vi "INSTRUMENTORDERSVotageAC5_6.vi"(0 "VISA资源名称":refnum<visa-resource-name>="DPO5054-C012667", 1 "打开通道":u16(ring) items=["CH1", "CH2", "CH3", "CH4"], 2 "关闭通道":u16(ring) items=["CH1", "CH2", "CH3", "CH4"], 3 "行索引":i32, 5 "错误输入（无错误）":errorcluster) -> (11 "FREQ":dbl, 13 "PERIOD":dbl, 14 "RMS":dbl, 15 "AMP":dbl, 16 "MAX":dbl, 17 "MIN":dbl, 18 "PK2PK":dbl, 19 "错误输出":errorcluster)   [LabVIEW 2014]
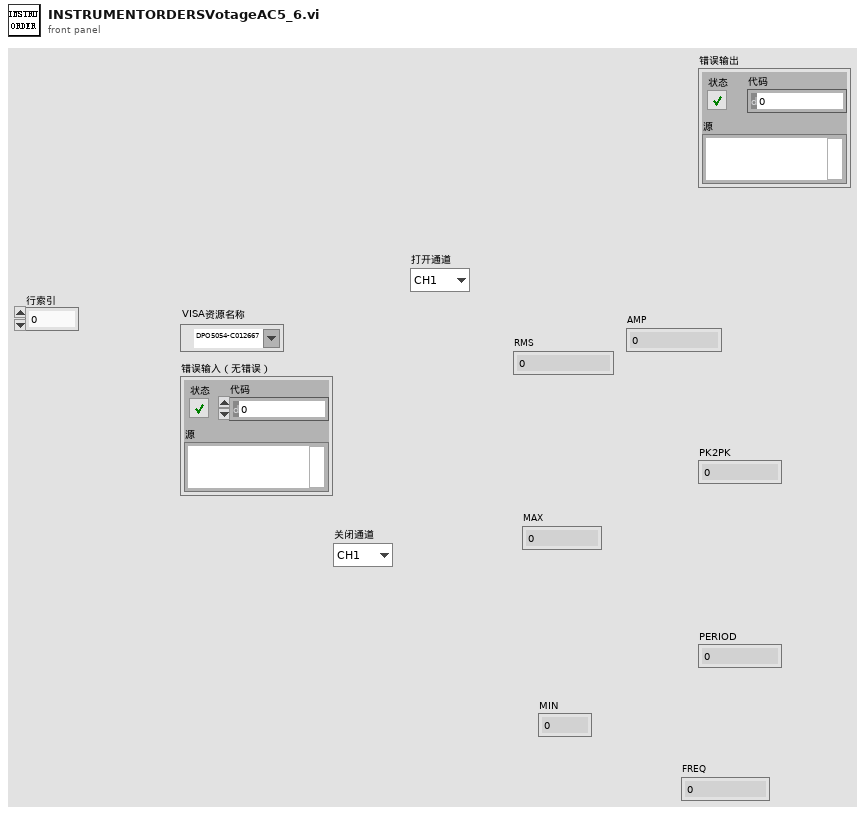
[diagram p1: front panel]
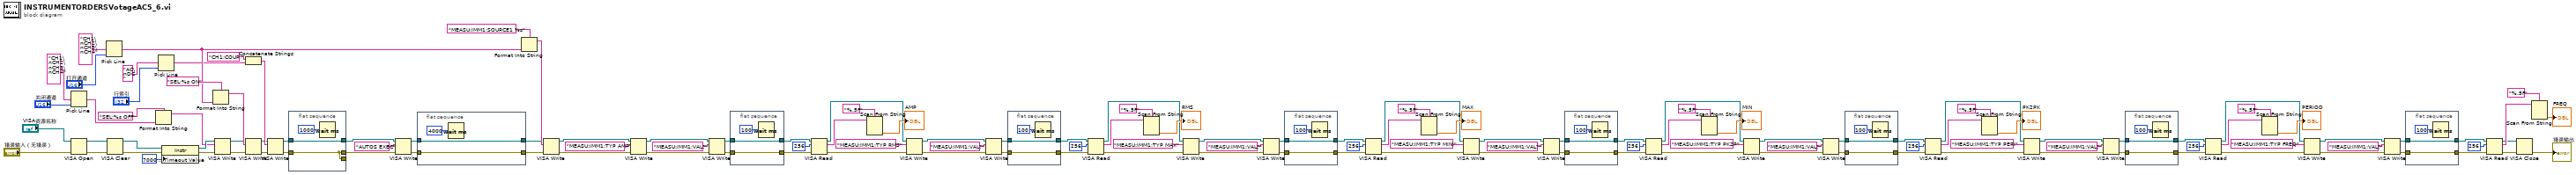
[diagram p0: block diagram]
diagram:
  n1 = Pick Line(multi-line string="CH1\nCH2\nCH3\nCH4" ("多行字符串"), line index="关闭通道") -> (output string=w113:string)  [unwired: 1 in]
  n2 = VISA Open(error in (no error)="错误输入（无错误）", VISA resource name="VISA资源名称") -> (VISA resource name=w139:refnum<visa-resource-name>, error out=w138:errorcluster)  [unwired: 3 in]
  n3 = Pick Line(multi-line string="CH1\nCH2\nCH3\nCH4" ("多行字符串"), line index="打开通道") -> (output string=w118:string)  [unwired: 1 in]
  n4 = VISA Clear(VISA resource name=w139, error in (no error)=w138) -> (VISA resource name out=w137:refnum<visa-resource-name>, error out=w136:errorcluster)
  n5 = Format Into String(format string="SEL:%s OFF" ("格式字符串"), w113) -> (resulting string=w109:string)  [unwired: 2 in, 1 out]
  n6 = Pick Line(multi-line string="AC\nDC", line index="行索引") -> (output string=w12:string)  [unwired: 1 in]
  n7 = property class="Instr"(reference=w137, error in=w136, "General Settings:Timeout Value"=u32 7000) -> (reference out=w115:refnum<visa-resource-name>, error out=w114:errorcluster)
  n8 = Format Into String(format string="SEL:%s ON" ("格式字符串"), w118) -> (resulting string=w117:string)  [unwired: 2 in, 1 out]
  n9 = VISA Write(VISA resource name=w115, write buffer=w109, error in (no error)=w114) -> (VISA resource name out=w108:refnum<visa-resource-name>, error out=w107:errorcluster)  [unwired: 1 out]
  n10 = Concatenate Strings("CH1:COUP " ("写入缓冲区"), w12) -> (w11:string)
  n11 = VISA Write(VISA resource name=w108, write buffer=w117, error in (no error)=w107) -> (VISA resource name out=w10:refnum<visa-resource-name>, error out=w9:errorcluster)  [unwired: 1 out]
  n12 = VISA Write(VISA resource name=w10, write buffer=w11, error in (no error)=w9) -> (VISA resource name out=w4:refnum<visa-resource-name>, error out=w3:errorcluster)  [unwired: 1 out]
  n13 = flat-sequence {
    tunnel: w4 -> [w142]
    tunnel: [w142] -> w2
    tunnel: w3 -> [w141]
    tunnel: [w141] -> _
    tunnel: [w141] -> w1
    frame #0 {
      n14 = Wait (ms)(milliseconds to wait=u32 1000 ("等待时间（毫秒）")) -> ()  [unwired: 1 out]
    }
  }
  n15 = VISA Write(VISA resource name=w2, write buffer="AUTOS EXEC" ("写入缓冲区"), error in (no error)=w1) -> (VISA resource name out=w8:refnum<visa-resource-name>, error out=w7:errorcluster)  [unwired: 1 out]
  n16 = flat-sequence {
    tunnel: w8 -> [w145]
    tunnel: [w145] -> w6
    tunnel: w7 -> [w144]
    tunnel: [w144] -> w5
    frame #0 {
      n17 = Wait (ms)(milliseconds to wait=u32 4000 ("等待时间（毫秒）")) -> ()  [unwired: 1 out]
    }
  }
  n18 = Format Into String(format string="MEASU:IMM1:SOURCE1 %s" ("格式字符串"), w118) -> (resulting string=w131:string)  [unwired: 2 in, 1 out]
  n19 = VISA Write(VISA resource name=w6, write buffer=w131, error in (no error)=w5) -> (VISA resource name out=w128:refnum<visa-resource-name>, error out=w127:errorcluster)  [unwired: 1 out]
  n20 = VISA Write(VISA resource name=w128, write buffer="MEASU:IMM1:TYP AMP" ("写入缓冲区"), error in (no error)=w127) -> (VISA resource name out=w124:refnum<visa-resource-name>, error out=w123:errorcluster)  [unwired: 1 out]
  n21 = VISA Write(VISA resource name=w124, write buffer="MEASU:IMM1:VAL?" ("写入缓冲区"), error in (no error)=w123) -> (VISA resource name out=w121:refnum<visa-resource-name>, error out=w120:errorcluster)  [unwired: 1 out]
  n22 = flat-sequence {
    tunnel: w121 -> [w148]
    tunnel: [w148] -> w126
    tunnel: w120 -> [w147]
    tunnel: [w147] -> w125
    frame #0 {
      n23 = Wait (ms)(milliseconds to wait=u32 100 ("等待时间（毫秒）")) -> ()  [unwired: 1 out]
    }
  }
  n24 = VISA Read(VISA resource name=w126, byte count=u32 256 ("字节总数"), error in (no error)=w125) -> (VISA resource name out=w30:refnum<visa-resource-name>, read buffer=w105:string, error out=w29:errorcluster)  [unwired: 1 out]
  n25 = Scan From String(format string="%.5F" ("格式字符串"), input string=w105) -> (output 1=→"AMP":dbl)  [unwired: 3 in, 3 out]
  n26 = VISA Write(VISA resource name=w30, write buffer="MEASU:IMM1:TYP RMS" ("写入缓冲区"), error in (no error)=w29) -> (VISA resource name out=w100:refnum<visa-resource-name>, error out=w101:errorcluster)  [unwired: 1 out]
  n27 = VISA Write(VISA resource name=w100, write buffer="MEASU:IMM1:VAL?" ("写入缓冲区"), error in (no error)=w101) -> (VISA resource name out=w92:refnum<visa-resource-name>, error out=w91:errorcluster)  [unwired: 1 out]
  n28 = flat-sequence {
    tunnel: w92 -> [w151]
    tunnel: [w151] -> w94
    tunnel: w91 -> [w150]
    tunnel: [w150] -> w95
    frame #0 {
      n29 = Wait (ms)(milliseconds to wait=u32 100 ("等待时间（毫秒）")) -> ()  [unwired: 1 out]
    }
  }
  n30 = VISA Read(VISA resource name=w94, byte count=u32 256 ("字节总数"), error in (no error)=w95) -> (VISA resource name out=w28:refnum<visa-resource-name>, read buffer=w96:string, error out=w27:errorcluster)  [unwired: 1 out]
  n31 = Scan From String(format string="%.5F" ("格式字符串"), input string=w96) -> (output 1=→"RMS":dbl)  [unwired: 3 in, 3 out]
  n32 = VISA Write(VISA resource name=w28, write buffer="MEASU:IMM1:TYP MAX" ("写入缓冲区"), error in (no error)=w27) -> (VISA resource name out=w81:refnum<visa-resource-name>, error out=w80:errorcluster)  [unwired: 1 out]
  n33 = VISA Write(VISA resource name=w81, write buffer="MEASU:IMM1:VAL?" ("写入缓冲区"), error in (no error)=w80) -> (VISA resource name out=w89:refnum<visa-resource-name>, error out=w90:errorcluster)  [unwired: 1 out]
  n34 = flat-sequence {
    tunnel: w89 -> [w154]
    tunnel: [w154] -> w87
    tunnel: w90 -> [w153]
    tunnel: [w153] -> w86
    frame #0 {
      n35 = Wait (ms)(milliseconds to wait=u32 100 ("等待时间（毫秒）")) -> ()  [unwired: 1 out]
    }
  }
  n36 = VISA Read(VISA resource name=w87, byte count=u32 256 ("字节总数"), error in (no error)=w86) -> (VISA resource name out=w26:refnum<visa-resource-name>, read buffer=w85:string, error out=w25:errorcluster)  [unwired: 1 out]
  n37 = Scan From String(format string="%.5F" ("格式字符串"), input string=w85) -> (output 1=→"MAX":dbl)  [unwired: 3 in, 3 out]
  n38 = VISA Write(VISA resource name=w26, write buffer="MEASU:IMM1:TYP MINI" ("写入缓冲区"), error in (no error)=w25) -> (VISA resource name out=w76:refnum<visa-resource-name>, error out=w77:errorcluster)  [unwired: 1 out]
  n39 = VISA Write(VISA resource name=w76, write buffer="MEASU:IMM1:VAL?" ("写入缓冲区"), error in (no error)=w77) -> (VISA resource name out=w68:refnum<visa-resource-name>, error out=w67:errorcluster)  [unwired: 1 out]
  n40 = flat-sequence {
    tunnel: w68 -> [w157]
    tunnel: [w157] -> w70
    tunnel: w67 -> [w156]
    tunnel: [w156] -> w71
    frame #0 {
      n41 = Wait (ms)(milliseconds to wait=u32 100 ("等待时间（毫秒）")) -> ()  [unwired: 1 out]
    }
  }
  n42 = VISA Read(VISA resource name=w70, byte count=u32 256 ("字节总数"), error in (no error)=w71) -> (VISA resource name out=w24:refnum<visa-resource-name>, read buffer=w72:string, error out=w23:errorcluster)  [unwired: 1 out]
  n43 = Scan From String(format string="%.5F" ("格式字符串"), input string=w72) -> (output 1=→"MIN":dbl)  [unwired: 3 in, 3 out]
  n44 = VISA Write(VISA resource name=w24, write buffer="MEASU:IMM1:TYP PK2P" ("写入缓冲区"), error in (no error)=w23) -> (VISA resource name out=w57:refnum<visa-resource-name>, error out=w56:errorcluster)  [unwired: 1 out]
  n45 = VISA Write(VISA resource name=w57, write buffer="MEASU:IMM1:VAL?" ("写入缓冲区"), error in (no error)=w56) -> (VISA resource name out=w65:refnum<visa-resource-name>, error out=w66:errorcluster)  [unwired: 1 out]
  n46 = flat-sequence {
    tunnel: w65 -> [w160]
    tunnel: [w160] -> w63
    tunnel: w66 -> [w159]
    tunnel: [w159] -> w62
    frame #0 {
      n47 = Wait (ms)(milliseconds to wait=u32 100 ("等待时间（毫秒）")) -> ()  [unwired: 1 out]
    }
  }
  n48 = VISA Read(VISA resource name=w63, byte count=u32 256 ("字节总数"), error in (no error)=w62) -> (VISA resource name out=w22:refnum<visa-resource-name>, read buffer=w61:string, error out=w21:errorcluster)  [unwired: 1 out]
  n49 = Scan From String(format string="%.5F" ("格式字符串"), input string=w61) -> (output 1=→"PK2PK":dbl)  [unwired: 3 in, 3 out]
  n50 = VISA Write(VISA resource name=w22, write buffer="MEASU:IMM1:TYP PERI" ("写入缓冲区"), error in (no error)=w21) -> (VISA resource name out=w52:refnum<visa-resource-name>, error out=w53:errorcluster)  [unwired: 1 out]
  n51 = VISA Write(VISA resource name=w52, write buffer="MEASU:IMM1:VAL?" ("写入缓冲区"), error in (no error)=w53) -> (VISA resource name out=w44:refnum<visa-resource-name>, error out=w43:errorcluster)  [unwired: 1 out]
  n52 = flat-sequence {
    tunnel: w44 -> [w163]
    tunnel: [w163] -> w46
    tunnel: w43 -> [w162]
    tunnel: [w162] -> w47
    frame #0 {
      n53 = Wait (ms)(milliseconds to wait=u32 100 ("等待时间（毫秒）")) -> ()  [unwired: 1 out]
    }
  }
  n54 = VISA Read(VISA resource name=w46, byte count=u32 256 ("字节总数"), error in (no error)=w47) -> (VISA resource name out=w20:refnum<visa-resource-name>, read buffer=w48:string, error out=w19:errorcluster)  [unwired: 1 out]
  n55 = Scan From String(format string="%.5F" ("格式字符串"), input string=w48) -> (output 1=→"PERIOD":dbl)  [unwired: 3 in, 3 out]
  n56 = VISA Write(VISA resource name=w20, write buffer="MEASU:IMM1:TYP FREQ" ("写入缓冲区"), error in (no error)=w19) -> (VISA resource name out=w33:refnum<visa-resource-name>, error out=w32:errorcluster)  [unwired: 1 out]
  n57 = VISA Write(VISA resource name=w33, write buffer="MEASU:IMM1:VAL?" ("写入缓冲区"), error in (no error)=w32) -> (VISA resource name out=w41:refnum<visa-resource-name>, error out=w42:errorcluster)  [unwired: 1 out]
  n58 = flat-sequence {
    tunnel: w41 -> [w166]
    tunnel: [w166] -> w39
    tunnel: w42 -> [w165]
    tunnel: [w165] -> w38
    frame #0 {
      n59 = Wait (ms)(milliseconds to wait=u32 100 ("等待时间（毫秒）")) -> ()  [unwired: 1 out]
    }
  }
  n60 = VISA Read(VISA resource name=w39, byte count=u32 256 ("字节总数"), error in (no error)=w38) -> (VISA resource name out=w18:refnum<visa-resource-name>, read buffer=w37:string, error out=w17:errorcluster)  [unwired: 1 out]
  n61 = VISA Close(VISA resource name=w18, error in (no error)=w17) -> (error out=→"错误输出":errorcluster)
  n62 = Scan From String(format string="%.5F" ("格式字符串"), input string=w37) -> (output 1=→"FREQ":dbl)  [unwired: 3 in, 3 out]
